vi "WFGConfigureReadBack.vi"(0 "object in":refnum<class "AD2_WFG_SDK.lvclass">, 2 "Ch":T1={"idxChannel"=0, "Settings out of range"=FALSE, "Carrier"={"Frequency (Hz)"=1000.0, "Amplitude (V)"=1.0, "Offset(V)"=0.0, "Symmetry(%) "=50.0, "Phase(Deg)"=0.0, "Function"=1, "Enable"=FALSE}, "Trigger"={"secRun(0=Cont)"=0.0, "secWait"=0.0, "cRepeat(0=inf)"=0, "Repeat Trigger"=FALSE, "TrigrSrc"=enum."trigrsrcNone"}, "FM Mod"={"Frequency (Hz)"=1000.0, "Amplitude (%)"=1.0, "Offset(V)"=0.0, "Symmetry(%) "=50.0, "Phase(Deg)"=0.0, "Function 2"=1, "Enable"=FALSE}} {"FM Mod"."Function 2" items=["DC"=0, "Sine"=1, "Square"=2, "Triangle"=3, "RampUp"=4, "RampDown"=5, "Noise"=6, "Pulse"=7, "Custom"=30]; "Carrier"."Function" items=["DC"=0, "Sine"=1, "Square"=2, "Triangle"=3, "RampUp"=4, "RampDown"=5, "Noise"=6, "Pulse"=7, "Custom"=30]}, 5 "error in (no error)":errorcluster) -> (14 "object out":refnum<class "AD2_WFG_SDK.lvclass">, 16 "Ch out":T1={"idxChannel"=0, "Settings out of range"=FALSE, "Carrier"={"Frequency (Hz)"=1000.0, "Amplitude (V)"=1.0, "Offset(V)"=0.0, "Symmetry(%) "=50.0, "Phase(Deg)"=0.0, "Function"=1, "Enable"=FALSE}, "Trigger"={"secRun(0=Cont)"=0.0, "secWait"=0.0, "cRepeat(0=inf)"=0, "Repeat Trigger"=FALSE, "TrigrSrc"=enum."trigrsrcNone"}, "FM Mod"={"Frequency (Hz)"=1000.0, "Amplitude (%)"=1.0, "Offset(V)"=0.0, "Symmetry(%) "=50.0, "Phase(Deg)"=0.0, "Function 2"=1, "Enable"=FALSE}} {"FM Mod"."Function 2" items=["DC"=0, "Sine"=1, "Square"=2, "Triangle"=3, "RampUp"=4, "RampDown"=5, "Noise"=6, "Pulse"=7, "Custom"=30]; "Carrier"."Function" items=["DC"=0, "Sine"=1, "Square"=2, "Triangle"=3, "RampUp"=4, "RampDown"=5, "Noise"=6, "Pulse"=7, "Custom"=30]}, 19 "error out":errorcluster)   [LabVIEW 2019, in "AD2_WFG_SDK.lvclass"]
uses:
  AD2_WFG_SDK.lvclass
  WFGCh.ctl
  AD2TriggerSources.ctl
  AD2_WFG_SDK.lvclass/AD2_WFG_SDK.ctl
  Olasdwf/Olasdwf.lvlib
  AD2_SDK_class/AD2_SDK.lvclass
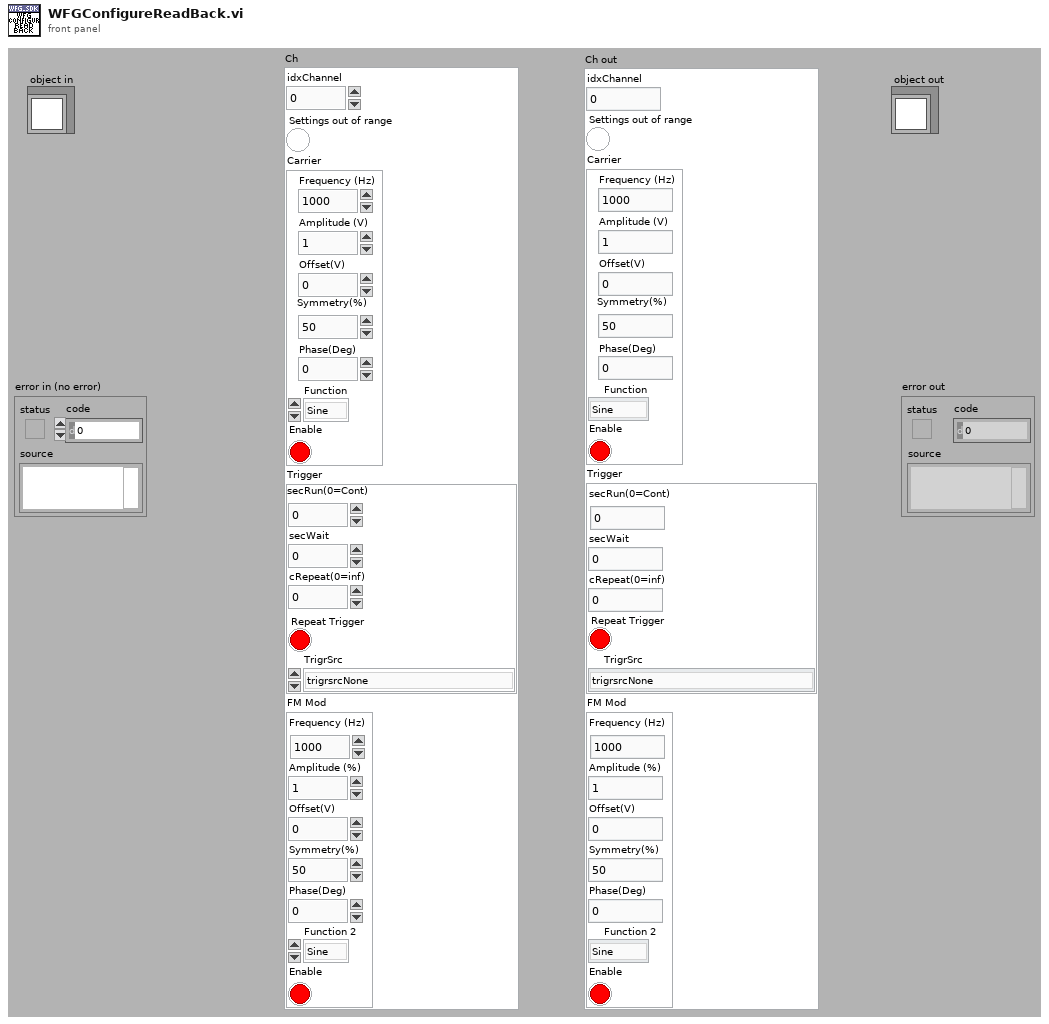
[diagram p1: front panel]
types:
  T1 = typedef "AD2_WFG_SDK.lvclass/WFGCh.ctl" = cluster{"idxChannel":i32, "Settings out of range":bool, "Carrier":cluster{"Frequency (Hz)":dbl, "Amplitude (V)":dbl, "Offset(V)":dbl, "Symmetry(%) ":dbl, "Phase(Deg)":dbl, "Function":u16, "Enable":bool}, "Trigger":cluster{"secRun(0=Cont)":dbl, "secWait":dbl, "cRepeat(0=inf)":i32, "Repeat Trigger":bool, "TrigrSrc":T2}, "FM Mod":cluster{"Frequency (Hz)":dbl, "Amplitude (%)":dbl, "Offset(V)":dbl, "Symmetry(%) ":dbl, "Phase(Deg)":dbl, "Function 2":u16, "Enable":bool}}
  T2 = typedef "AD2_SDK.lvclass/AD2TriggerSources.ctl" = enum8{"trigrsrcNone", "trigsrcPC", "trigsrcDetectorAnalogIn", "trigsrcDetectorDigitalIn", "trigsrcAnalogIn", "trigsrcDigitalIn", "trigsrcDigitalOut", "trigsrcAnalogOut1", "trigsrcAnalogOut2", "trigsrcAnalogOut3", "trigsrcAnalogOut4", "trigsrcExternal1", "trigsrcExternal2", "trigsrcExternal3", "trigsrcExternal4", ""}
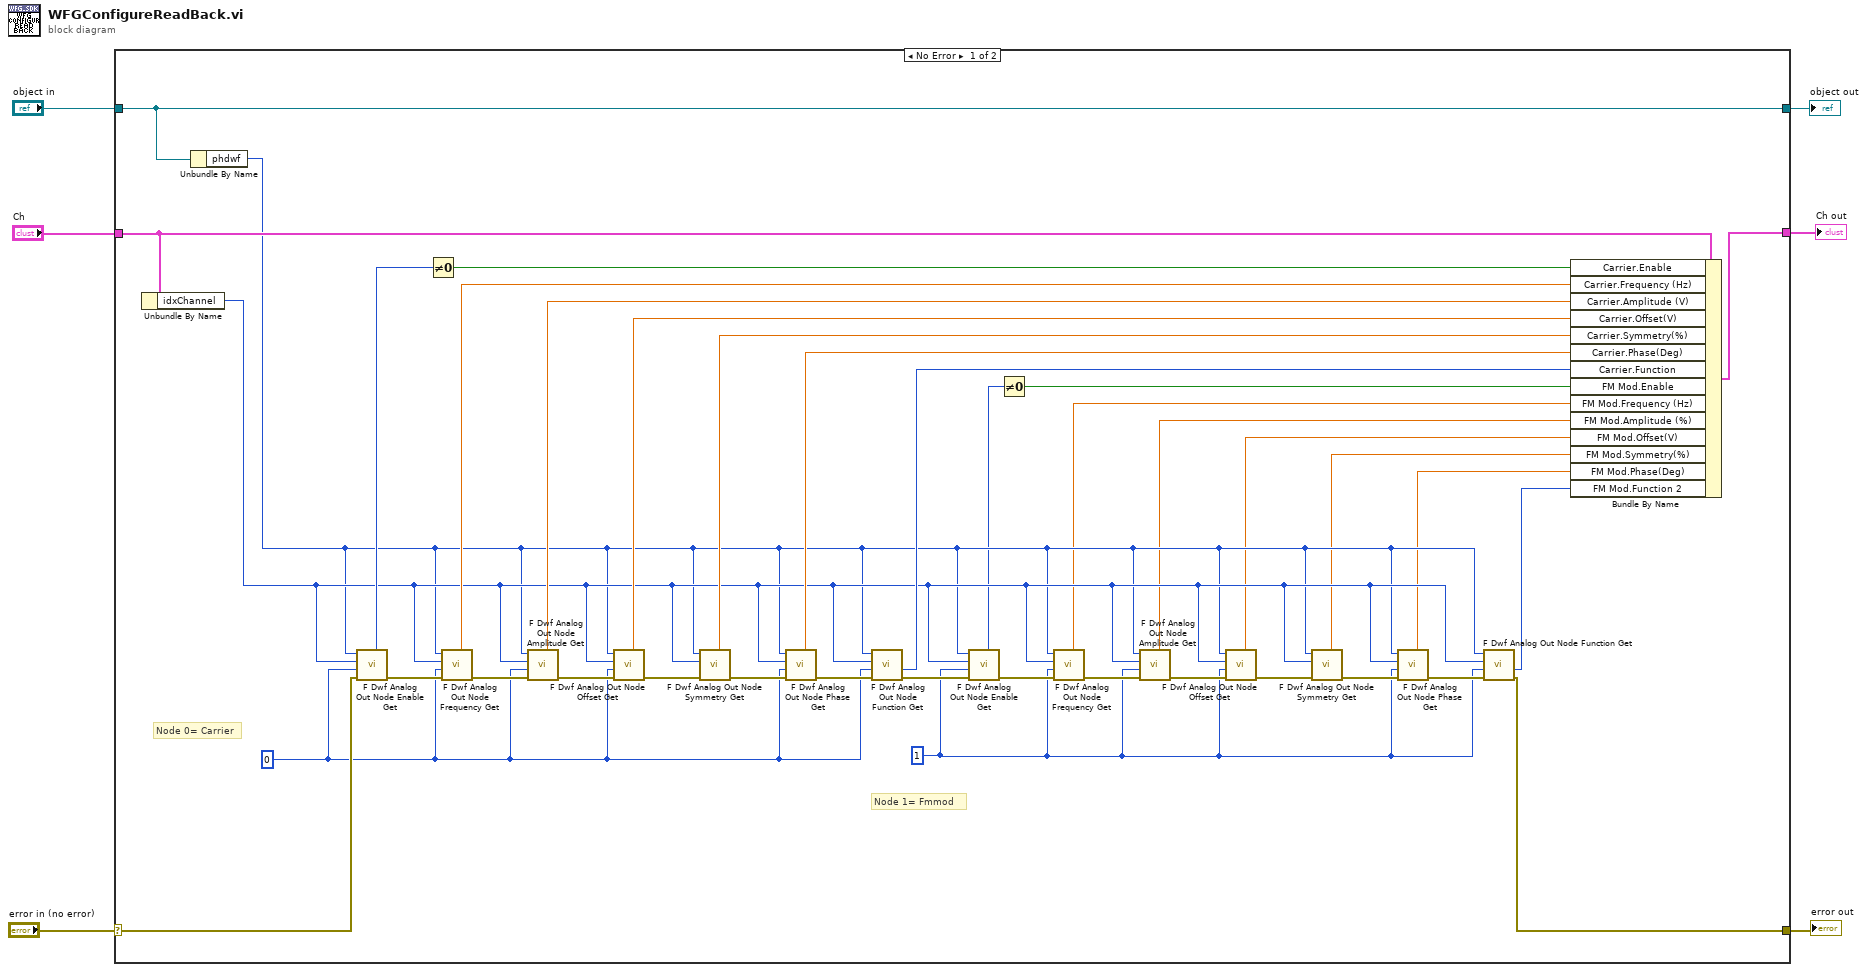
[diagram p0: block diagram]
diagram:
  n1 = case shown="No Error" "error in (no error)" {
    selector: "error in (no error)" -> [w28 w46]
    tunnel: [w13 w46] -> w5
    tunnel: [w44 w45] -> w3
    tunnel: "object in" -> [w44 w45]
    tunnel: "Ch" -> [w29 _]
    tunnel: [w27 _] -> w1
    frame No Error {
      w18 = 1 ("node")
      w26 = 0 ("node")
      # "Node 1= Fmmod"
      # "Node 0= Carrier"
      n2 = Unbundle By Name(w29) -> ("idxChannel"=w17:i32)
      n3 = Unbundle By Name(w44) -> ("phdwf"=w16:i32)
      n4 = call "F Dwf Analog Out Node Enable Get.vi"("error in (no error)"=w28, "node"=w26, "idxChannel"=w17, "hdwf"=w16) -> ("error out"=w30:errorcluster, "pfEnable out"=w36:i32)  [unwired: 5 in, 1 out]
      n5 = Not Equal To 0?(x=w36) -> (x != 0?=w35:bool)
      n6 = call "F Dwf Analog Out Node Frequency Get.vi"("error in (no error)"=w30, "node"=w26, "idxChannel"=w17, "hdwf"=w16) -> ("error out"=w31:errorcluster, "phzFrequency out"=w37:dbl)  [unwired: 5 in, 1 out]
      n7 = call "F Dwf Analog Out Node Amplitude Get.vi"("error in (no error)"=w31, "node"=w26, "idxChannel"=w17, "hdwf"=w16) -> ("error out"=w32:errorcluster, "pvAmplitude out"=w38:dbl)  [unwired: 5 in, 1 out]
      n8 = call "F Dwf Analog Out Node Offset Get.vi"("error in (no error)"=w32, "node"=w26, "idxChannel"=w17, "hdwf"=w16) -> ("error out"=w33:errorcluster, "pvOffset out"=w39:dbl)  [unwired: 5 in, 1 out]
      n9 = call "F Dwf Analog Out Node Symmetry Get.vi"("error in (no error)"=w33, "idxChannel"=w17, "hdwf"=w16) -> ("error out"=w34:errorcluster, "ppercentageSymmetry out"=w40:dbl)  [unwired: 6 in, 1 out]
      n10 = call "F Dwf Analog Out Node Phase Get.vi"("error in (no error)"=w34, "node"=w26, "idxChannel"=w17, "hdwf"=w16) -> ("error out"=w41:errorcluster, "pdegreePhase out"=w43:dbl)  [unwired: 5 in, 1 out]
      n11 = call "F Dwf Analog Out Node Function Get.vi"("error in (no error)"=w41, "node"=w26, "idxChannel"=w17, "hdwf"=w16) -> ("error out"=w19:errorcluster, "pfunc"=w42:u8)  [unwired: 5 in, 1 out]
      n12 = call "F Dwf Analog Out Node Enable Get.vi"("error in (no error)"=w19, "node"=w18, "idxChannel"=w17, "hdwf"=w16) -> ("error out"=w20:errorcluster, "pfEnable out"=w15:i32)  [unwired: 5 in, 1 out]
      n13 = Not Equal To 0?(x=w15) -> (x != 0?=w14:bool)
      n14 = call "F Dwf Analog Out Node Frequency Get.vi"("error in (no error)"=w20, "node"=w18, "idxChannel"=w17, "hdwf"=w16) -> ("error out"=w21:errorcluster, "phzFrequency out"=w12:dbl)  [unwired: 5 in, 1 out]
      n15 = call "F Dwf Analog Out Node Amplitude Get.vi"("error in (no error)"=w21, "node"=w18, "idxChannel"=w17, "hdwf"=w16) -> ("error out"=w22:errorcluster, "pvAmplitude out"=w11:dbl)  [unwired: 5 in, 1 out]
      n16 = call "F Dwf Analog Out Node Offset Get.vi"("error in (no error)"=w22, "node"=w18, "idxChannel"=w17, "hdwf"=w16) -> ("error out"=w23:errorcluster, "pvOffset out"=w10:dbl)  [unwired: 5 in, 1 out]
      n17 = call "F Dwf Analog Out Node Symmetry Get.vi"("error in (no error)"=w23, "idxChannel"=w17, "hdwf"=w16) -> ("error out"=w24:errorcluster, "ppercentageSymmetry out"=w9:dbl)  [unwired: 6 in, 1 out]
      n18 = call "F Dwf Analog Out Node Phase Get.vi"("error in (no error)"=w24, "node"=w18, "idxChannel"=w17, "hdwf"=w16) -> ("error out"=w25:errorcluster, "pdegreePhase out"=w8:dbl)  [unwired: 5 in, 1 out]
      n19 = call "F Dwf Analog Out Node Function Get.vi"("error in (no error)"=w25, "node"=w18, "idxChannel"=w17, "hdwf"=w16) -> ("error out"=w13:errorcluster, "pfunc"=w7:u8)  [unwired: 5 in, 1 out]
      n20 = Bundle By Name(cluster=w29, "Carrier.Enable"=w35, "Carrier.Frequency (Hz)"=w37, "Carrier.Amplitude (V)"=w38, "Carrier.Offset(V)"=w39, "Carrier.Symmetry(%)"=w40, "Carrier.Phase(Deg)"=w43, "Carrier.Function"=w42, "FM Mod.Enable"=w14, "FM Mod.Frequency (Hz)"=w12, "FM Mod.Amplitude (%)"=w11, "FM Mod.Offset(V)"=w10, "FM Mod.Symmetry(%)"=w9, "FM Mod.Phase(Deg)"=w8, "FM Mod.Function 2"=w7) -> (w27:T1)
    }
    frame Error {
    }
  }
  "error out" <- w5
  "object out" <- w3
  "Ch out" <- w1
